vi "DC Demo - CpivRamp - With AchSelect.vi"() -> ()   [LabVIEW 2012]
uses:
  DC Demo States.ctl
panel:
  in  "Ach Select":i32(ring) items=["BNC", "PSTAT", "CAPSTAT", "THERMO", "GND"]
  in  "Scan Rate":sgl=0.1 format="%_3f"
  in  "Final Voltage":sgl=1.0 format="%^_3e"
  in  "Initial Voltage":sgl format="%^_3e"
  out "event callback refnum":refnum<k27>
  out "Waveform Chart":sgl[][](graph)=[[0.99694026], [0.0009995501]]
  out "Section":string="PCI4300-32059"
  out "Signal":refnum<k7>
  in  "Sample Rate":sgl=0.5 format="%.3f"
  in  "GAMRYCOMLib.IGamrySignal":refnum<k7>
  out "Dtaq":refnum<k7>
  out "Pstat":refnum<k7>
  out "Device List":refnum<k7>
  out "Data Acquisition Complete":bool=TRUE
  in  "GAMRYCOMLib.IGamrySignalRamp":refnum<k7>
  in  "GAMRYCOMLib.IGamryDtaqCpiv":refnum<k7>
  in  "GAMRYCOMLib.IGamryPstat":refnum<k7>
  in  "GAMRYCOMLib.IGamryDeviceList":refnum<k7>
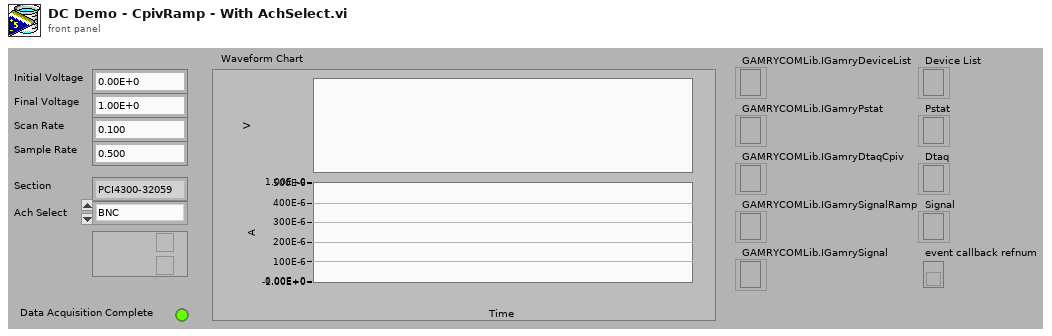
[diagram p1: front panel]
types:
  T1 = typedef "DC Demo States.ctl" = enum16{"Initialize Variables", "Initialize Pstat", "Initialize Dtaq", "Initialize Signal", "Set Signal", "Take Data", "Cleanup", "Stop"}
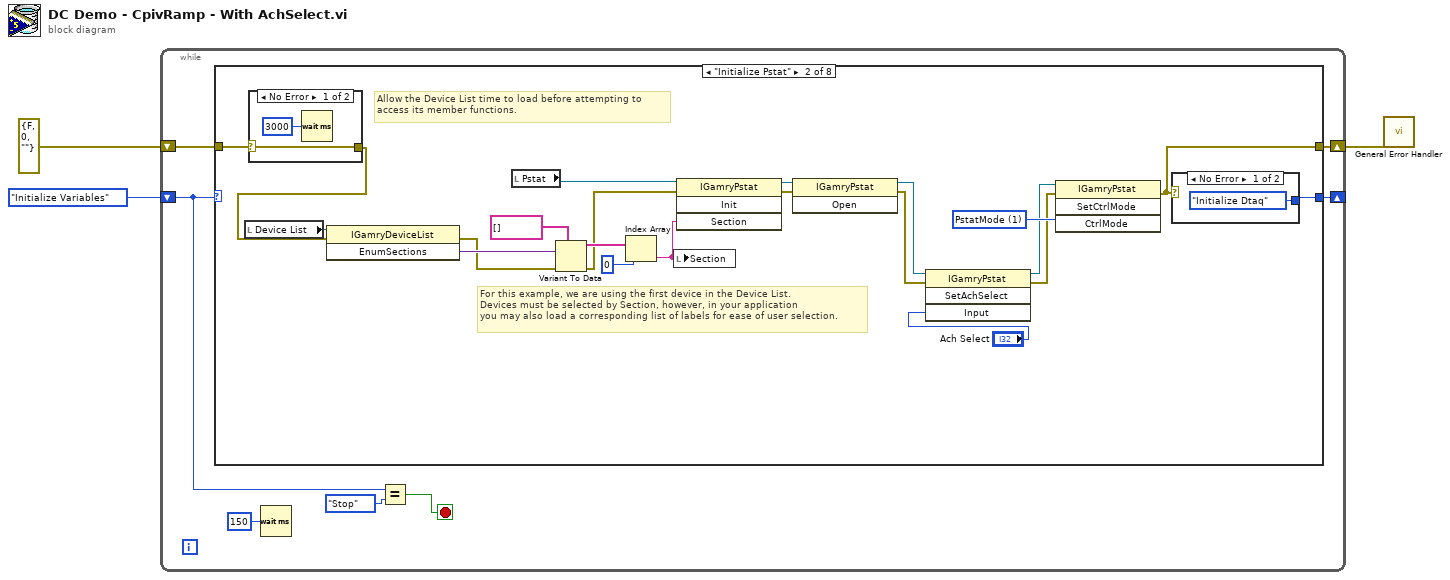
[diagram p0: block diagram]
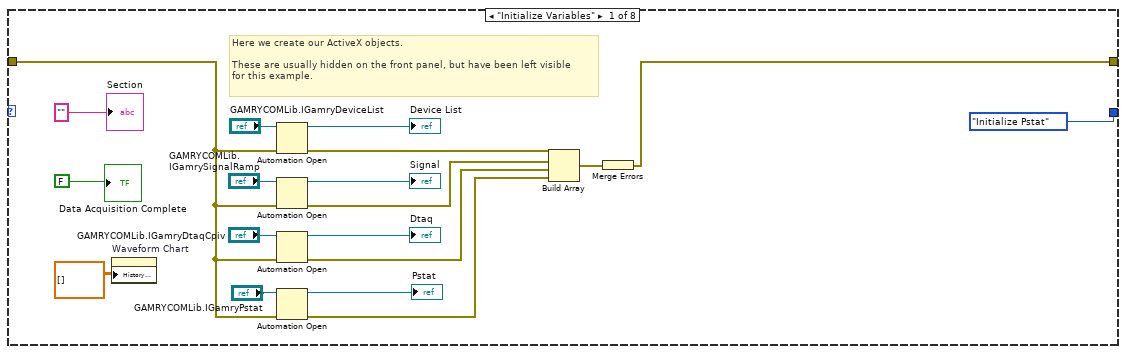
[diagram p2: hidden frame]
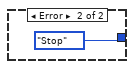
[diagram p4: hidden frame]
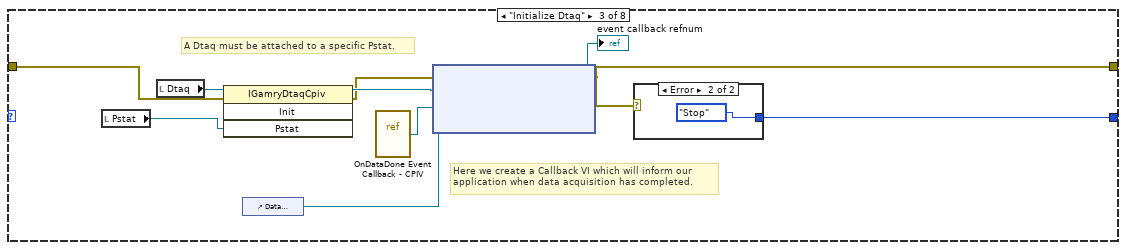
[diagram p5: hidden frame]
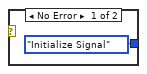
[diagram p6: hidden frame]
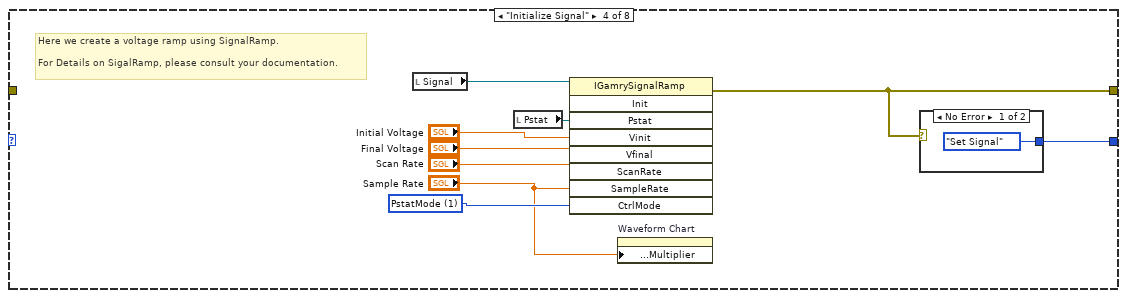
[diagram p7: hidden frame]
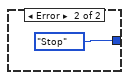
[diagram p8: hidden frame]
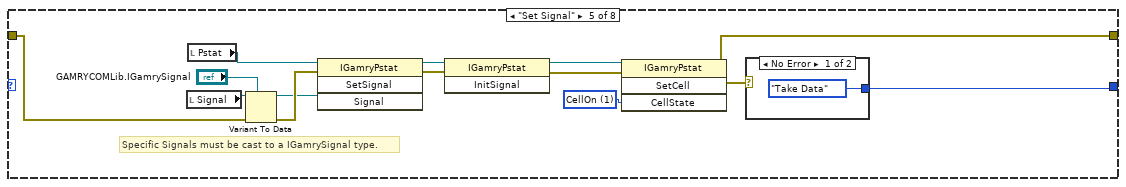
[diagram p9: hidden frame]
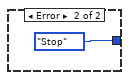
[diagram p10: hidden frame]
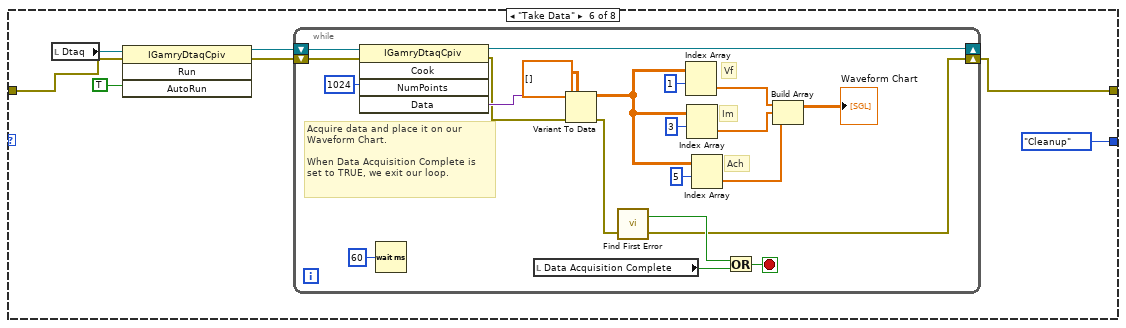
[diagram p11: hidden frame]
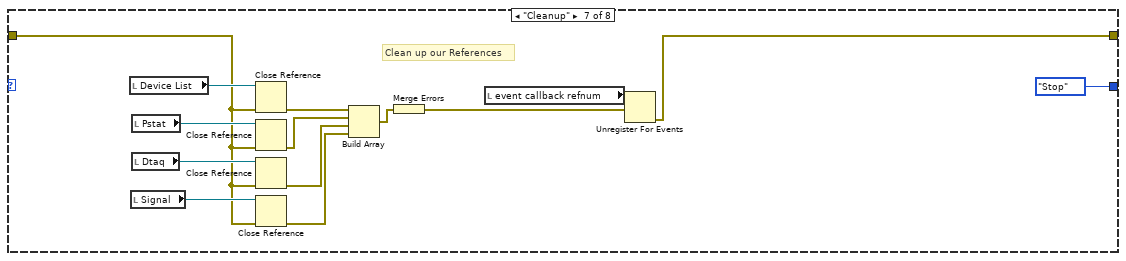
[diagram p12: hidden frame]
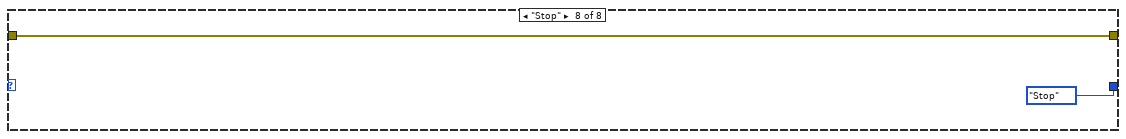
[diagram p13: hidden frame]
diagram:
  n1 = while {
    shift-right: [w7] -> _
    shift-left: DC_Demo_States."Initialize Variables" ("DC Demo States") -> [w8]
    shift-right: [w4] -> w2
    shift-left: errorcluster {"status"=FALSE, "code"=0, "source"=""} ("error in (no error)") -> [w5]
    stop <- w9 stop-if-true
    n2 = case shown="\"Initialize Pstat\"" w8 {
      tunnel: [DC_Demo_States."Initialize Pstat" ("DC Demo States") w47 w61 w76 w87 DC_Demo_States."Cleanup" ("DC Demo States") DC_Demo_States."Stop" ("DC Demo States") DC_Demo_States."Stop" ("DC Demo States")] -> w7
      tunnel: w5 -> [w13 w36 w59 _ w84 w95 w122 w136]
      tunnel: [w15 w41 w58 w74 w83 w94 w123 w136] -> w4
      frame "Initialize Variables" {
        # "Here we create our ActiveX objects.\n\nThese are usually hidden on the front panel, but have been left visible\nfor this example."
        n3 = property on="Waveform Chart" class="WFChart (strict)"("History Data"=sgl[][] []) -> ()  [unwired: 2 in, 2 out]
        n4 = Automation Open(error in (no error)=w13, Automation Refnum="GAMRYCOMLib.IGamryDeviceList") -> (Automation Refnum=→"Device List":refnum<k7>, error out=w20:errorcluster)  [unwired: 2 in]
        n5 = Automation Open(error in (no error)=w13, Automation Refnum="GAMRYCOMLib.IGamrySignalRamp") -> (Automation Refnum=→"Signal":refnum<k7>, error out=w19:errorcluster)  [unwired: 2 in]
        n6 = Automation Open(error in (no error)=w13, Automation Refnum="GAMRYCOMLib.IGamryDtaqCpiv") -> (Automation Refnum=→"Dtaq":refnum<k7>, error out=w18:errorcluster)  [unwired: 2 in]
        n7 = Automation Open(error in (no error)=w13, Automation Refnum="GAMRYCOMLib.IGamryPstat") -> (Automation Refnum=→"Pstat":refnum<k7>, error out=w17:errorcluster)  [unwired: 2 in]
        n8 = Build Array(w20, w19, w18, w17) -> (w16:errorcluster[])
        n9 = Merge Errors(w16) -> (w15:errorcluster)
        "Data Acquisition Complete" <- FALSE
        "Section" <- "" ("Section")
      }
      frame "Initialize Pstat" {
        w50 = 1 items=["GstatMode", "PstatMode", "ZRAMode", "FRAMode"] ("CtrlMode")
        # "For this example, we are using the first device in the Device List.\nDevices must be selected by Section, however, in your application\nyou may also load a corresponding list of labels for ease of user selection."
        # "Allow the Device List time to load before attempting to \naccess its member functions."
        n10 = local read "Device List"() -> (w40:refnum<k7>)
        n11 = case shown="No Error" w36 {
          selector: w36 -> [w51 w53]
          tunnel: [w51 w53] -> w35
          frame No Error {
            n12 = Wait (ms)(milliseconds to wait=u32 3000) -> ()  [unwired: 1 out]
          }
          frame Error {
          }
        }
        n13 = invoke class="IGamryDeviceList" method="EnumSections"(reference=w40, error in=w35) -> (error out=w38:errorcluster, "EnumSections"=w39:variant)  [unwired: 1 in, 1 out]
        n14 = local read "Pstat"() -> (w43:refnum<k7>)
        n15 = Variant To Data(error in=w38, type=string[] [], Variant=w39) -> (data=w45:string[], error out=w37:errorcluster)
        n16 = Index Array(array=w45, index=0) -> (element=w42:string)
        n17 = local write "Section"(w42) -> ()
        n18 = invoke class="IGamryPstat" method="Init"(reference=w43, error in=w37, "Section"=w42) -> (reference out=w49:refnum<k7>, error out=w48:errorcluster)  [unwired: 1 in, 2 out]
        n19 = invoke class="IGamryPstat" method="Open"(reference=w49, error in=w48) -> (reference out=w31:refnum<k7>, error out=w33:errorcluster)  [unwired: 1 in, 1 out]
        n20 = invoke class="IGamryPstat" method="SetAchSelect"(reference=w31, error in=w33, "Input"="Ach Select") -> (reference out=w30:refnum<k7>, error out=w34:errorcluster)  [unwired: 1 in, 2 out]
        n21 = invoke class="IGamryPstat" method="SetCtrlMode"(reference=w30, error in=w34, "CtrlMode"=w50) -> (error out=w41:errorcluster)  [unwired: 1 in, 3 out]
        n22 = case shown="No Error" w41 {
          tunnel: [DC_Demo_States."Initialize Dtaq" ("DC Demo States") DC_Demo_States."Stop" ("DC Demo States")] -> w47
          frame No Error {
          }
          frame Error {
          }
        }
      }
      frame "Initialize Dtaq" {
        # "A Dtaq must be attached to a specific Pstat."
        # "Here we create a Callback VI which will inform our\napplication when data acquisition has completed."
        n23 = local read "Pstat"() -> (w56:refnum<k7>)
        n24 = local read "Dtaq"() -> (w60:refnum<k7>)
        n25 = invoke class="IGamryDtaqCpiv" method="Init"(reference=w60, error in=w59, "Pstat"=w56) -> (reference out=w63:refnum<k7>, error out=w62:errorcluster)  [unwired: 1 in, 2 out]
        n26 = control-ref of="Data Acquisition Complete"() -> (w65:refnum<vi>)
        n27 = vi-ref "OnDataDone Event Callback - CPIV.vi"() -> ("vi reference"=w64:refnum<vi>)
        n28 = node(w62, w63, w64, w65) -> (→"event callback refnum":refnum<k27>, w58:errorcluster)  [unwired: 1 in]
        n29 = case shown="Error" w58 {
          tunnel: [DC_Demo_States."Initialize Signal" ("DC Demo States") DC_Demo_States."Stop" ("DC Demo States")] -> w61
          frame No Error {
          }
          frame Error {
          }
        }
      }
      frame "Initialize Signal" {
        w70 = 1 items=["GstatMode", "PstatMode", "ZRAMode", "FRAMode"] ("CtrlMode")
        # "Here we create a voltage ramp using SignalRamp.\n\nFor Details on SigalRamp, please consult your documentation."
        n30 = local read "Signal"() -> (w75:refnum<k7>)
        n31 = local read "Pstat"() -> (w68:refnum<k7>)
        n32 = invoke class="IGamrySignalRamp" method="Init"(reference=w75, "Pstat"=w68, "Vinit"="Initial Voltage", "Vfinal"="Final Voltage", "ScanRate"="Scan Rate", "SampleRate"="Sample Rate", "CtrlMode"=w70) -> (error out=w74:errorcluster)  [unwired: 2 in, 8 out]
        n33 = property on="Waveform Chart" class="WFChart (strict)"("X Scale.Offset and Multiplier:Multiplier"="Sample Rate") -> ()  [unwired: 2 in, 2 out]
        n34 = case shown="No Error" w74 {
          tunnel: [DC_Demo_States."Set Signal" ("DC Demo States") DC_Demo_States."Stop" ("DC Demo States")] -> w76
          frame No Error {
          }
          frame Error {
          }
        }
      }
      frame "Set Signal" {
        w90 = 1 items=["CellOff", "CellOn"] ("CellState")
        # "Specific Signals must be cast to a IGamrySignal type."
        n35 = local read "Signal"() -> (w86:refnum<k7>)
        n36 = local read "Pstat"() -> (w85:refnum<k7>)
        n37 = Variant To Data(error in=w84, type="GAMRYCOMLib.IGamrySignal", Variant=w86) -> (data=w88:refnum<k7>, error out=w91:errorcluster)
        n38 = invoke class="IGamryPstat" method="SetSignal"(reference=w85, error in=w91, "Signal"=w88) -> (reference out=w82:refnum<k7>, error out=w81:errorcluster)  [unwired: 1 in, 2 out]
        n39 = invoke class="IGamryPstat" method="InitSignal"(reference=w82, error in=w81) -> (reference out=w80:refnum<k7>, error out=w79:errorcluster)  [unwired: 1 in, 1 out]
        n40 = invoke class="IGamryPstat" method="SetCell"(reference=w80, error in=w79, "CellState"=w90) -> (error out=w83:errorcluster)  [unwired: 1 in, 3 out]
        n41 = case shown="No Error" w83 {
          tunnel: [DC_Demo_States."Take Data" ("DC Demo States") DC_Demo_States."Stop" ("DC Demo States")] -> w87
          frame No Error {
          }
          frame Error {
          }
        }
      }
      frame "Take Data" {
        n42 = local read "Dtaq"() -> (w99:refnum<k7>)
        n43 = invoke class="IGamryDtaqCpiv" method="Run"(reference=w99, error in=w95, "AutoRun"=TRUE) -> (reference out=w97:refnum<k7>, error out=w96:errorcluster)  [unwired: 1 in, 2 out]
        n44 = while {
          shift-right: [w111] -> w94
          shift-left: w96 -> [w120]
          shift-right: [w110] -> _
          shift-left: w97 -> [w121]
          stop <- w112 stop-if-true
          # "Ach"
          # "Im"
          # "Vf"
          # "Acquire data and place it on our\nWaveform Chart.\n\nWhen Data Acquisition Complete is\nset to TRUE, we exit our loop."
          n45 = invoke class="IGamryDtaqCpiv" method="Cook"(reference=w121, error in=w120, "NumPoints"=1024) -> (reference out=w110:refnum<k7>, error out=w116:errorcluster, "Data"=w117:variant)  [unwired: 2 in, 2 out]
          n46 = Wait (ms)(milliseconds to wait=u32 60) -> ()  [unwired: 1 out]
          n47 = local read "Data Acquisition Complete"() -> (w113:bool)
          n48 = Variant To Data(error in=w116, type=sgl[][] [], Variant=w117) -> (data=w102:sgl[][], error out=w115:errorcluster)
          n49 = call <vilib>:"Find First Error.vi"("error in (no error)"=w115) -> ("error out"=w111:errorcluster, "error?"=w114:bool)  [unwired: 3 in]
          n50 = Index Array(array=w102, index (row)=1) -> (element=w107:sgl[])  [unwired: 1 in]
          n51 = Index Array(array=w102, index (row)=3) -> (element=w108:sgl[])  [unwired: 1 in]
          n52 = Index Array(array=w102, index (row)=5) -> (element=w101:sgl[])  [unwired: 1 in]
          n53 = Or(x=w114, y=w113) -> (x .or. y?=w112:bool)
          n54 = Build Array(w107, w108, w101) -> (→"Waveform Chart":sgl[][])
        }
      }
      frame "Cleanup" {
        # "Clean up our References"
        n55 = local read "Device List"() -> (w134:refnum<k7>)
        n56 = local read "Signal"() -> (w131:refnum<k7>)
        n57 = local read "Pstat"() -> (w133:refnum<k7>)
        n58 = local read "Dtaq"() -> (w132:refnum<k7>)
        n59 = Close Reference(reference=w134, error in (no error)=w122) -> (error out=w130:errorcluster)
        n60 = Close Reference(reference=w133, error in (no error)=w122) -> (error out=w129:errorcluster)
        n61 = Close Reference(reference=w132, error in (no error)=w122) -> (error out=w128:errorcluster)
        n62 = Close Reference(reference=w131, error in (no error)=w122) -> (error out=w127:errorcluster)
        n63 = Build Array(w130, w129, w128, w127) -> (w126:errorcluster[])
        n64 = Merge Errors(w126) -> (w124:errorcluster)
        n65 = local read "event callback refnum"() -> (w125:refnum<k27>)
        n66 = Unregister For Events(event registration refnum=w125, error in=w124) -> (error out=w123:errorcluster)
      }
      frame "Stop" {
      }
    }
    n67 = Wait (ms)(milliseconds to wait=u32 150) -> ()  [unwired: 1 out]
    n68 = Equal?(x=w8, y=DC_Demo_States."Stop" ("DC Demo States")) -> (x = y?=w9:bool)
  }
  n69 = call <vilib>:"General Error Handler.vi"("error in (no error)"=w2) -> ()  [unwired: 10 in, 5 out]
